vi "Get Players.vi"(11 "Game in":refnum<class "Game.lvclass">) -> (2 "Players":refnum<class "User.lvclass">[](array[class]))   [LabVIEW 2020, in "Conditum-Example.lvlib" / "Game.lvclass"]
uses:
  Game.lvclass
  Conditum/Columns/Entity Collection/Entity Collection.lvclass
  User/User.lvclass
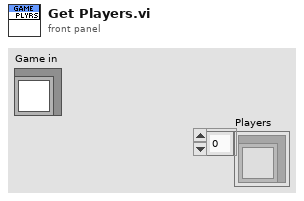
[diagram p1: front panel]
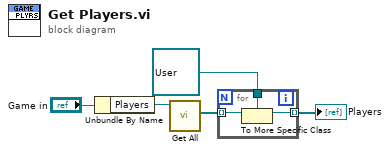
[diagram p0: block diagram]
diagram:
  n1 = Unbundle By Name("Game in") -> ("Players"=w4:refnum<class "Entity Collection.lvclass">)
  n2 = call "Get All.vi"("Entity Collection in"=w4) -> ("Entities"=w3:refnum<class "Entity.lvclass">[])  [unwired: 10 in]
  n3 = for {
    tunnel: w3 -> [w8] mode=indexing
    tunnel: refnum<class "User.lvclass"> refnum ("Conditum-Example.lvlib:User.lvclass") -> [w7]
    tunnel: [w6] -> w1 mode=indexing
    n4 = To More Specific Class(target class=w7, reference=w8) -> (specific class reference=w6:refnum<class "User.lvclass">)  [unwired: 1 in, 1 out]
  }
  "Players" <- w1
